vi "CurrentLocation.vi"(1 "Longitude":string, 2 "Latitude":string) -> (0 "marker":string)   [LabVIEW 2015]
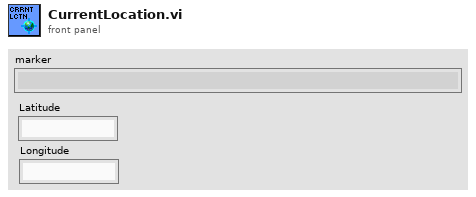
[diagram p1: front panel]
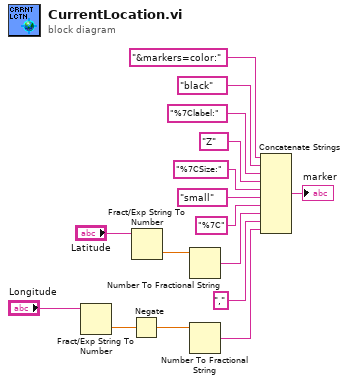
[diagram p0: block diagram]
diagram:
  n1 = Fract/Exp String To Number(string="Longitude") -> (number=w5:dbl)  [unwired: 3 in, 1 out]
  n2 = Negate(x=w5) -> (-x=w4:dbl)
  n3 = Fract/Exp String To Number(string="Latitude") -> (number=w3:dbl)  [unwired: 3 in, 1 out]
  n4 = Number To Fractional String(number=w3) -> (F-format string=w1:string)  [unwired: 3 in]
  n5 = Number To Fractional String(number=w4) -> (F-format string=w6:string)  [unwired: 3 in]
  n6 = Concatenate Strings("&markers=color:", "black" ("Color"), "%7Clabel:" ("string"), "Z" ("Character"), "%7CSize:" ("string"), "small" ("Size"), "%7C" ("string"), w1, ",", w6) -> (→"marker":string)
